vi "Update VS channels (interaction data).vi"(9 "receiveInteraction in":T1, 10 "hla map helpers in":T6, 11 "values in":dbl[](array[numeric])) -> (1 "receiveInteraction out":T1, 2 "hla map helpers out":T6, 3 "values out":dbl[](array[numeric]))   [LabVIEW 2019, in "HLA Custom Device Engine.lvlib"]
uses:
  HLA Custom Device Engine.lvlib
  _typedefs/RThlaMapHelpers.ctl
  _typedefs/map_in_interaction.ctl
  _typedefs/map_interaction_value.ctl
  _typedefs/map_attr_param_data.ctl
  _typedefs/map_object.ctl
  _typedefs/map_object_key.ctl
  _typedefs/map_object_value.ctl
  _typedefs/map_object_instance.ctl
  _typedefs/map_object_instance_value.ctl
  _typedefs/map_object_vs_instance.ctl
  _typedefs/map_out_vs_ch_interaction.ctl
  _typedefs/receiveInteraction_type.ctl
  _typedefs/interaction_info_received_type.ctl
  emea-ni-adg-hla-lv/src/library/typedefs/TransportationType.ctl
  emea-ni-adg-hla-lv/src/library/typedefs/OrderType.ctl
  _typedefs/dataElement_type.ctl
  Data Encoding_Decoding/HLA Data Conversion.lvlib
  emea-ni-adg-hla-lv/src/library/openrti_rti1516eLv.lvlib
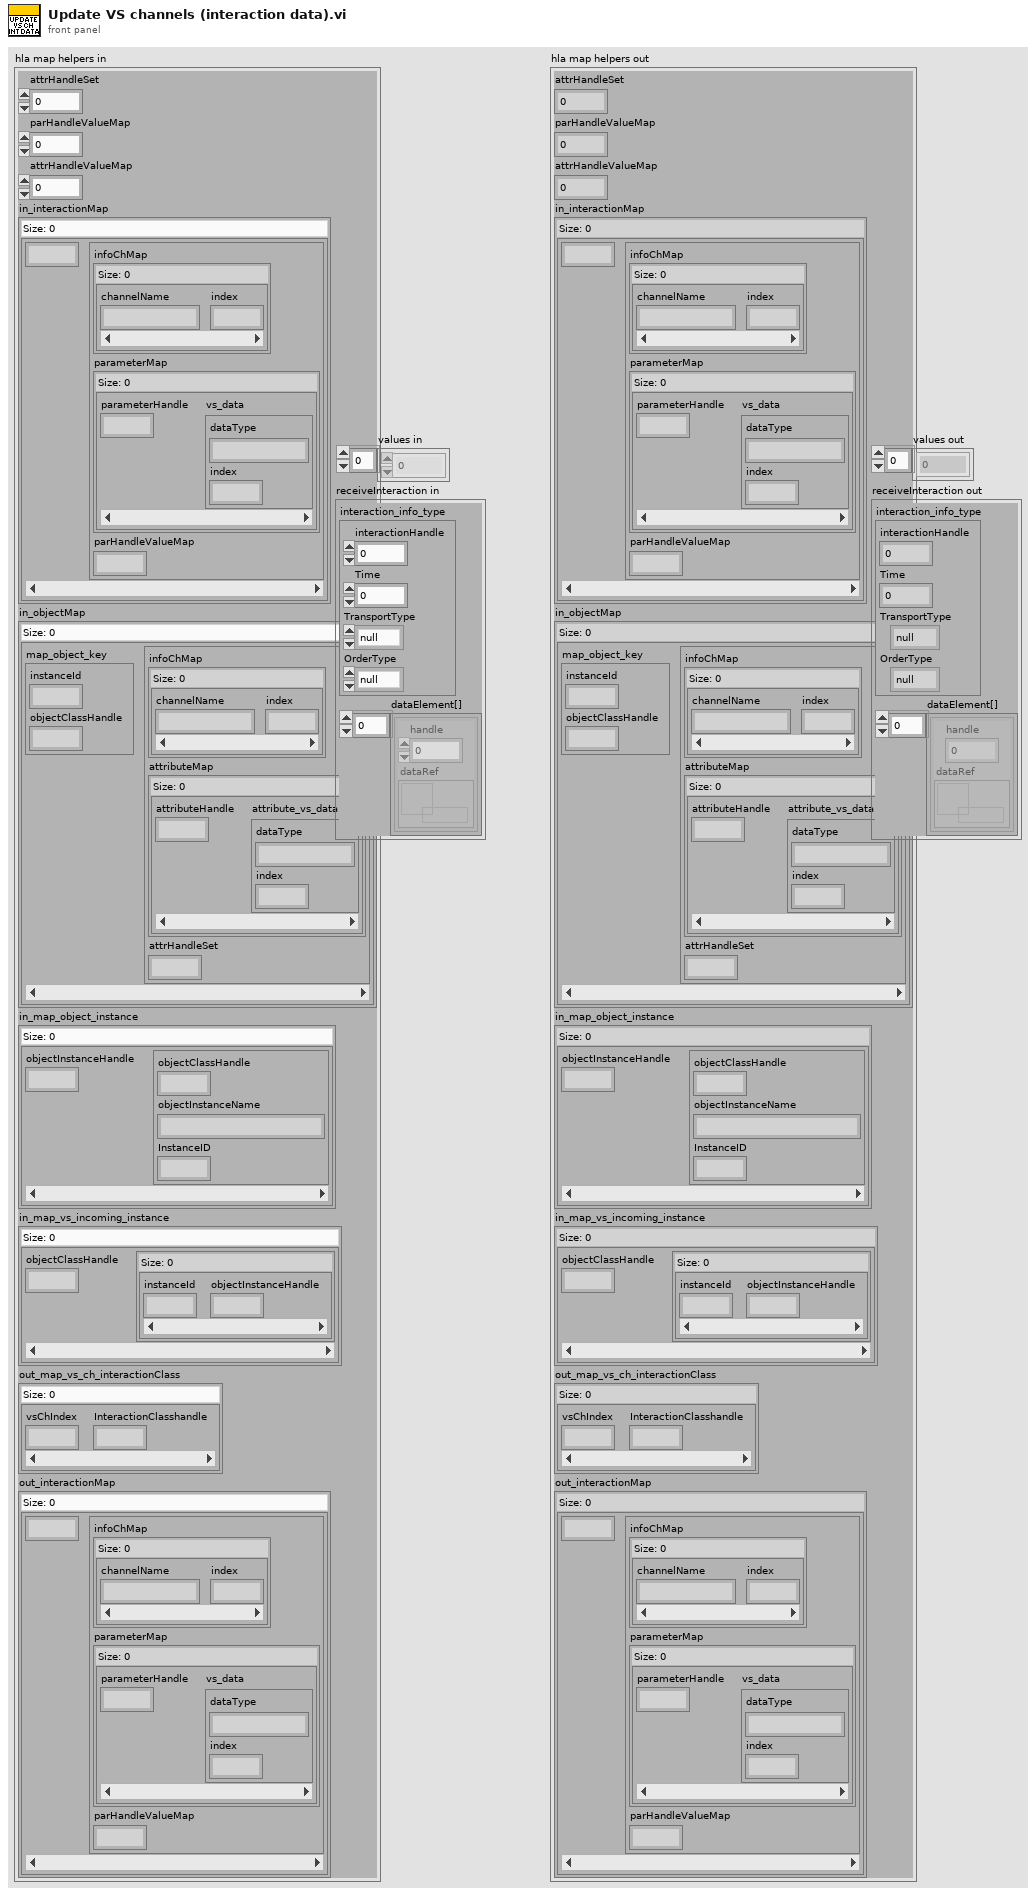
[diagram p1: front panel]
types:
  T1 = typedef "HLA Custom Device Engine.lvlib/receiveInteraction_type.ctl" = cluster{"interaction_info_type":T2, "dataElement[]":T5[]}
  T2 = typedef "HLA Custom Device Engine.lvlib/interaction_info_received_type.ctl" = cluster{"interactionHandle":u64, "Time":u32, "TransportType":T3, "OrderType":T4}
  T3 = typedef "openrti_rti1516eLv.lvlib/TransportationType.ctl" = enum32{"null", "RELIABLE", "BEST_EFFORT"}
  T4 = typedef "openrti_rti1516eLv.lvlib/OrderType.ctl" = enum32{"null", "RECEIVE", "TIMESTAMP"}
  T5 = typedef "HLA Custom Device Engine.lvlib/dataElement_type.ctl" = cluster{"handle":u64, "dataRef":refnum<data-value>}
  T6 = typedef "HLA Custom Device Engine.lvlib/RThlaMapHelpers.ctl" = cluster{"attrHandleSet":u64, "parHandleValueMap":u64, "attrHandleValueMap":u64, "in_interactionMap":T7, "in_objectMap":T10, "in_map_object_instance":T13, "in_map_vs_incoming_instance":T15, "out_map_vs_ch_interactionClass":T16, "out_interactionMap":T7}
  T7 = typedef "HLA Custom Device Engine.lvlib/map_in_interaction.ctl" = map{u64, T8}
  T8 = typedef "HLA Custom Device Engine.lvlib/map_interaction_value.ctl" = cluster{"infoChMap":map{string, i32}, "parameterMap":map{u64, T9}, "parHandleValueMap":u64}
  T9 = typedef "HLA Custom Device Engine.lvlib/map_attr_param_data.ctl" = cluster{"dataType":string, "index":i32}
  T10 = typedef "HLA Custom Device Engine.lvlib/map_object.ctl" = map{T11, T12}
  T11 = typedef "HLA Custom Device Engine.lvlib/map_object_key.ctl" = cluster{"instanceId":i32, "objectClassHandle":u64}
  T12 = typedef "HLA Custom Device Engine.lvlib/map_object_value.ctl" = cluster{"infoChMap":map{string, i32}, "attributeMap":map{u64, T9}, "attrHandleSet":u64}
  T13 = typedef "HLA Custom Device Engine.lvlib/map_object_instance.ctl" = map{u64, T14}
  T14 = typedef "HLA Custom Device Engine.lvlib/map_object_instance_value.ctl" = cluster{"objectClassHandle":u64, "objectInstanceName":string, "InstanceID":i32}
  T15 = typedef "HLA Custom Device Engine.lvlib/map_object_vs_instance.ctl" = map{u64, map{i32, u64}}
  T16 = typedef "HLA Custom Device Engine.lvlib/map_out_vs_ch_interaction.ctl" = map{i32, u64}
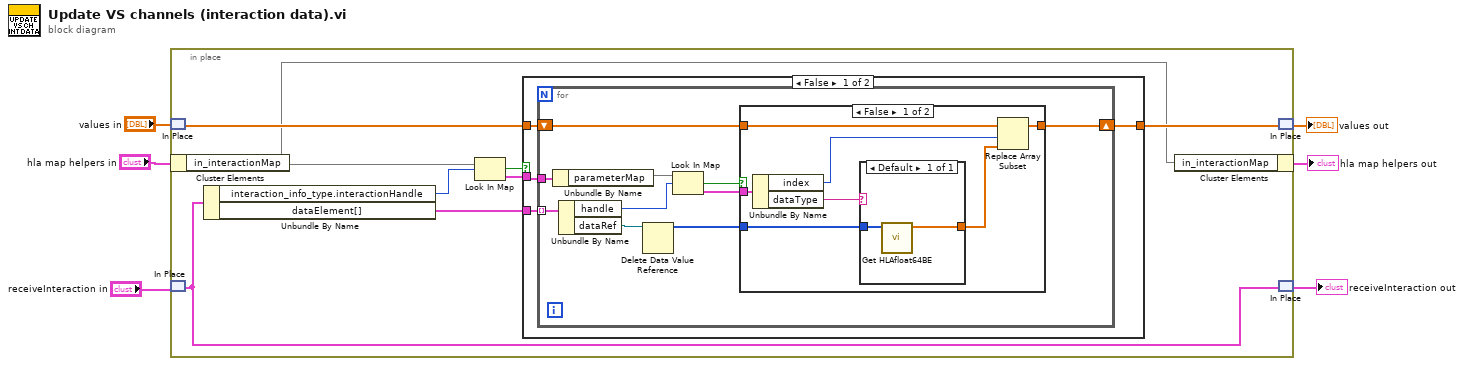
[diagram p0: block diagram]
diagram:
  n1 = in-place {
    n2 = in-place-match #1("values in") -> (w11:dbl[])
    n3 = in-place-cluster #2("hla map helpers in") -> ("in_interactionMap"=w9:T7)
    n4 = in-place-match #3("receiveInteraction in") -> (w7:T1)
    n5 = Unbundle By Name(w7) -> ("interaction_info_type.interactionHandle"=w14:u64, "dataElement[]"=w8:T5[])
    n6 = Look In Map(map=w9, key=w14) -> (key not found?=w13:bool, value=w12:T8)  [unwired: 1 in]
    n7 = case shown="False" w13 {
      tunnel: [w18 w39] -> w10
      tunnel: w12 -> [w17 _]
      tunnel: w11 -> [w16 w39]
      tunnel: w8 -> [w15 _]
      frame False {
        n8 = for {
          tunnel: w17 -> [w25]
          tunnel: w15 -> [w22] mode=indexing
          shift-right: [w27] -> w18
          shift-left: w16 -> [w23]
          n9 = Unbundle By Name(w25) -> ("parameterMap"=w24:map{u64, T9})
          n10 = Unbundle By Name(w22) -> ("handle"=w21:u64, "dataRef"=w20:refnum<data-value>)
          n11 = Delete Data Value Reference(data value reference=w20) -> (data value=w19:u8[])  [unwired: 1 in, 1 out]
          n12 = Look In Map(map=w24, key=w21) -> (key not found?=w28:bool, value=w26:T9)  [unwired: 1 in]
          n13 = case shown="False" w28 {
            tunnel: [w35 w38] -> w27
            tunnel: w26 -> [w32 _]
            tunnel: w23 -> [w30 w38]
            tunnel: w19 -> [w29 _]
            frame False {
              n14 = Unbundle By Name(w32) -> ("index"=w33:i32, "dataType"=w34:string)
              n15 = case shown="Default" w34 {
                tunnel: [w37] -> w31
                tunnel: w29 -> [w36]
                frame Default {
                  n16 = call "Get HLAfloat64BE.vi"("raw data in"=w36) -> ("eu data out"=w37:dbl[])  [unwired: 9 in, 1 out]
                }
              }
              n17 = Replace Array Subset(array=w30, new element=w31, index=w33) -> (w35:dbl[])
            }
            frame True {
            }
          }
        }
      }
      frame True {
      }
    }
    n18 = in-place-cluster #2("in_interactionMap"=w9) -> (→"hla map helpers out":T6)
    n19 = in-place-match #1(w10) -> (→"values out":dbl[])
    n20 = in-place-match #3(w7) -> (→"receiveInteraction out":T1)
  }
